vi "A_W_extracter.vi"() -> ()   [LabVIEW 2014]
uses:
  <vilib>/Utility/file.llb/Read From Spreadsheet File (DBL).vi
panel:
  out "Selected(Num)":i16[](array[numeric])
  in  "Spectrogram":path
  out "W":dbl[][](array[numeric])
  out "A":dbl[][](array[numeric])
  in  "Variables":T1={"s_verbose"=enum."On", "displayInterval"=1.0, "displayMode"=enum."On", "sampleSize"=1.0, "guess"=[[1.0]], "initState"=enum."rand", "maxFinetune"=100.0, "maxNumIteration"=100.0, "epsilon"=0.0001, "stabilization"=enum."On", "myy"=1.0, "a1"=1.0, "a2"=1.0, "finetune"=enum."off", "g"=enum."pow3", "approach"=enum."symm"}
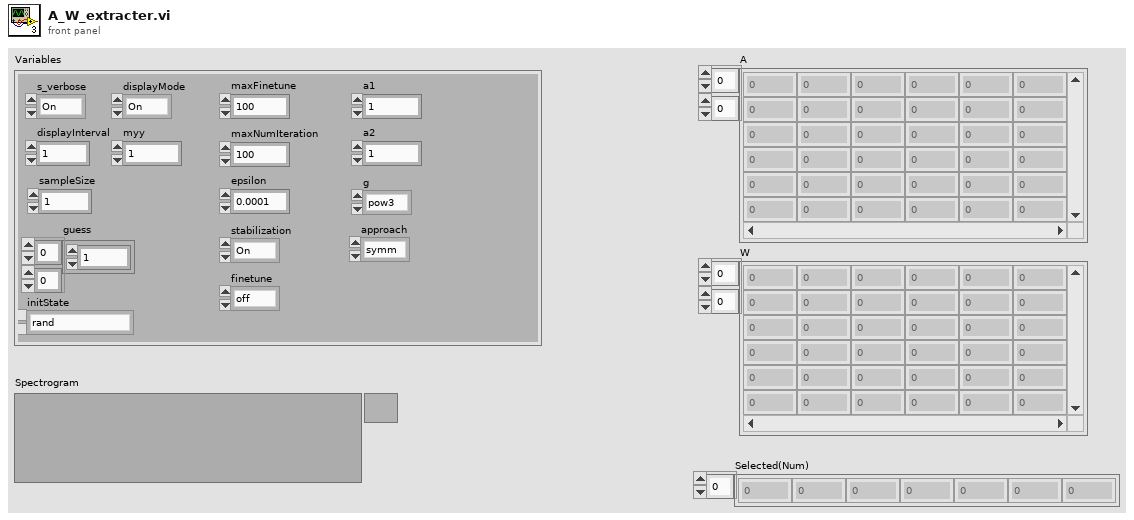
[diagram p1: front panel]
types:
  T1 = cluster{"s_verbose":enum16{"Off", "On"}, "displayInterval":dbl, "displayMode":enum16{"Off", "On"}, "sampleSize":dbl, "guess":dbl[][], "initState":enum16{"rand", "guess"}, "maxFinetune":dbl, "maxNumIteration":dbl, "epsilon":dbl, "stabilization":enum16{"Off", "On"}, "myy":dbl, "a1":dbl, "a2":dbl, "finetune":enum16{"pow3", "tanh", "gauss", "skew", "off"}, "g":enum16{"pow3", "tanh", "gauss", "skew"}, "approach":enum16{"symm", "delf"}}
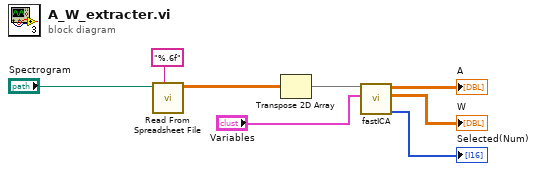
[diagram p0: block diagram]
diagram:
  n1 = call-poly <vilib>:"Read From Spreadsheet File.vi"("format (%.3f)"="%.6f", "file path (dialog if empty)"="Spectrogram") -> ("all rows"=w4:dbl[][])  [unwired: 5 in, 4 out]
  n2 = Transpose 2D Array(2D array=w4) -> (transposed array=w8:dbl[][])
  n3 = call "fastICA.vi"("Variables"="Variables", "Input Data (X)"=w8) -> ("Selected(Num)"=→"Selected(Num)":i16[], "W"=→"W":dbl[][], "A"=→"A":dbl[][])  [unwired: 7 in]
